vi "Instrument.Oxford1820.GetPublicEvents.vi"(8 "error in (no error)":errorcluster, 11 "Instrument.Oxford1820 in":refnum<class "Instrument.Oxford1820.lvclass">) -> (0 "error out":errorcluster, 2 "OI1820 Public Events":T1, 3 "Instrument.Oxford1820 out":refnum<class "Instrument.Oxford1820.lvclass">)   [LabVIEW 2016, in "Instrument.Oxford1820.lvclass"]
uses:
  Instrument.Oxford1820.lvclass
  Typedefs/PublicEvents--Cluster.ctl
  Typedefs/PublicEvents--Instrument.Oxford1820.ProcessStatus.ctl
  Instrument.Oxford1820.lvclass/Instrument.Oxford1820.ctl
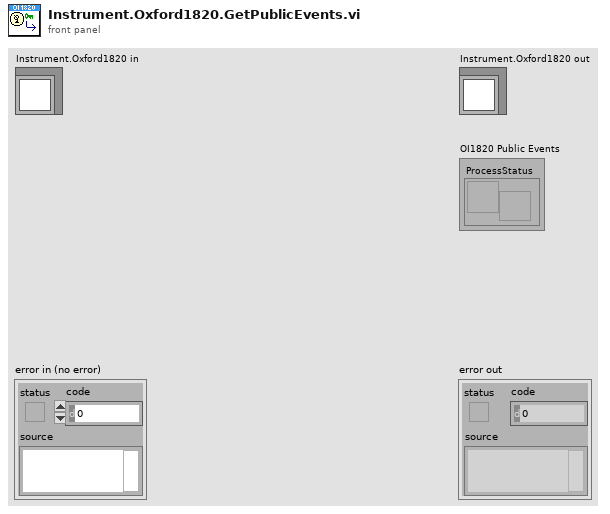
[diagram p1: front panel]
types:
  T1 = typedef "Instrument.Oxford1820.lvclass/PublicEvents--Cluster.ctl" = cluster{"ProcessStatus":refnum<user-event>}
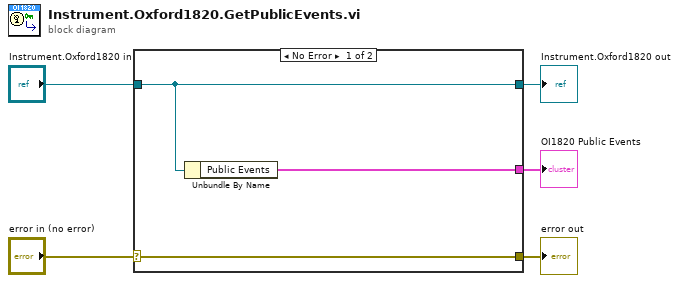
[diagram p0: block diagram]
diagram:
  n1 = case shown="No Error" "error in (no error)" {
    selector: "error in (no error)" -> [w8 w9]
    tunnel: [w8 w9] -> w4
    tunnel: [w7 w10] -> w2
    tunnel: "Instrument.Oxford1820 in" -> [w7 w10]
    tunnel: [w6 _] -> w1
    frame No Error {
      n2 = Unbundle By Name(w7) -> ("Public Events"=w6:T1)
    }
    frame Error {
    }
  }
  "error out" <- w4
  "Instrument.Oxford1820 out" <- w2
  "OI1820 Public Events" <- w1
